vi "Read.vi"(8 "error in (no error)":errorcluster, 11 "HP 3457A in":refnum<class "HP 3457A.lvclass">) -> (0 "error out":errorcluster, 1 "Unit":string, 2 "Measure":dbl, 3 "HP 3457A out":refnum<class "HP 3457A.lvclass">, 4 "Channel":i32)   [LabVIEW 2020, in "HP 3457A.lvclass"]
uses:
  HP 3457A.lvclass
  C:/Sandbox/Git_Sandbox/WiSpry Test Framework source code (LV20)/WiSpry Test Framework/Instruments/Digital Multimeter/Digital Multimeter.lvclass
  C:/Sandbox/Git_Sandbox/WiSpry Test Framework source code (LV20)/WiSpry Test Framework/Instruments/Instrument.lvclass
  Instrument.lvclass/Instrument.ctl
  Digital Multimeter.lvclass/Digital Multimeter.ctl
  Instrument.lvclass
  Digital Multimeter.lvclass
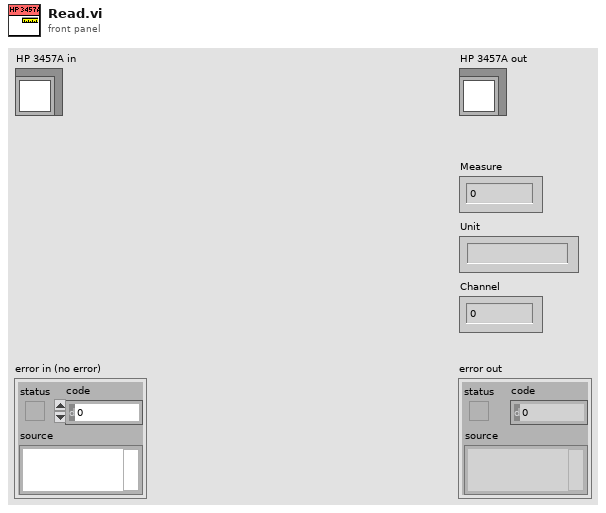
[diagram p1: front panel]
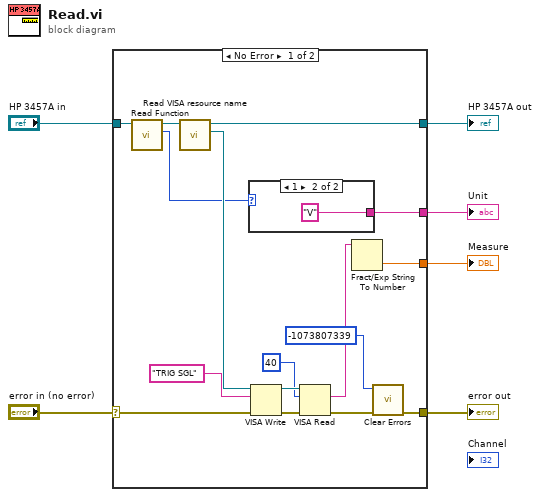
[diagram p0: block diagram]
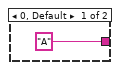
[diagram p2: hidden frame]
diagram:
  n1 = case shown="No Error" "error in (no error)" {
    selector: "error in (no error)" -> [w17 w26]
    tunnel: "HP 3457A in" -> [w9 w25]
    tunnel: [w15 w26] -> w3
    tunnel: [w22 w25] -> w4
    tunnel: [w12 _] -> w2
    tunnel: [w11 _] -> w1
    frame No Error {
      n2 = call "Read Function.vi"("Digtal Multimeter in"=w9) -> ("Function"=w7:u16, "Digtal Multimeter out"=w8:refnum<class "HP 3457A.lvclass">)  [unwired: 9 in]
      n3 = call "Read VISA resource name.vi"("Instrument in"=w8) -> ("VISA resource name"=w16:refnum<visa-resource-name>, "Instrument out"=w22:refnum<class "HP 3457A.lvclass">)  [unwired: 9 in]
      n4 = case shown="1" w7 {
        tunnel: ["A" "V"] -> w11
        frame 0, Default {
        }
        frame 1 {
        }
      }
      n5 = VISA Write(VISA resource name=w16, write buffer="TRIG SGL", error in (no error)=w17) -> (VISA resource name out=w21:refnum<visa-resource-name>, error out=w20:errorcluster)  [unwired: 1 out]
      n6 = VISA Read(VISA resource name=w21, byte count=u32 40, error in (no error)=w20) -> (read buffer=w13:string, error out=w14:errorcluster)  [unwired: 2 out]
      n7 = Fract/Exp String To Number(string=w13) -> (number=w12:dbl)  [unwired: 3 in, 1 out]
      n8 = call <vilib>:"Clear Errors.vi"("error in (no error)"=w14, "specific error code to clear (0: all)"=-1073807339) -> ("error out"=w15:errorcluster)  [unwired: 4 in, 1 out]
    }
    frame Error {
    }
  }
  "error out" <- w3
  "HP 3457A out" <- w4
  "Measure" <- w2
  "Unit" <- w1
